vi "Read - Asynchronous.vi"(8 "error in":errorcluster, 11 "Serial IO in":refnum<class "Serial IO.lvclass">) -> (0 "error out":errorcluster, 2 "read buffer":string, 3 "Serial IO out":refnum<class "Serial IO.lvclass">)   [LabVIEW 2015, in "Serial IO.lvclass"]
doc: "Read asynchronously from the serial port. Requires no prior write."
uses:
  Serial IO.lvclass
  Serial IO.lvclass/Serial IO.ctl
  <vilib>/Platform/TimedLoop/XDataNode/timing_clust.ctl
  <vilib>/Platform/TimedLoop/XDataNode/nitl_modes.ctl
  <vilib>/Platform/TimedLoop/XDataNode/wakeup.ctl
  <vilib>/Platform/TimedLoop/XDataNode/XDataNode.xnode
  <vilib>/Platform/TimedLoop/XDataNode/XDNodeRunTimeDep.lvlib
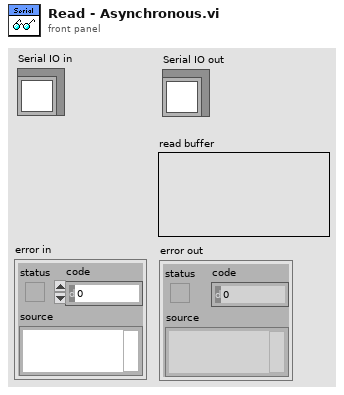
[diagram p1: front panel]
types:
  T1 = typedef "XDNodeRunTimeDep.lvlib/timing_clust.ctl" = cluster{"Expected End [f-1]":u64, "Actual End [f-1]":u64, "Finished Late? [f-1]":bool, "Expected End [i-1]":u64, "Actual End [i-1]":u64, "Finished Late? [i-1]":bool, "Expected Start [i]":u64, "Actual Start [i]":u64, "Expected Start [f]":u64, "Actual Start [f]":u64, "Source Name":string, "Structure Name":string, "Period":i64, "Deadline":i64, "Offset":i64, "Start":i64, "Priority":i32, "Timeout":i32, "Mode":T2, "Wakeup Reason":T3, "Error":errorcluster, "Source Type":string, "Secondary Source Type":string, "Global End Time":u64, "Global Start Time":u64, "Frame Duration":u64, "Iteration Duration":u64, "Assigned CPU":i32, "I/O Scan Engine Mode":u32}
  T2 = typedef "XDNodeRunTimeDep.lvlib/nitl_modes.ctl" = enum32{"No Change", "Process missed periods, maintain original phase", "Discard missed periods, maintain original phase", "Process missed periods, ignore original phase", "Discard missed periods, ignore original phase"}
  T3 = typedef "XDNodeRunTimeDep.lvlib/wakeup.ctl" = enum32{"Normal", "Aborted", "Asynchronous wakeup", "Timing source error", "Timed loop error", "Timeout"}
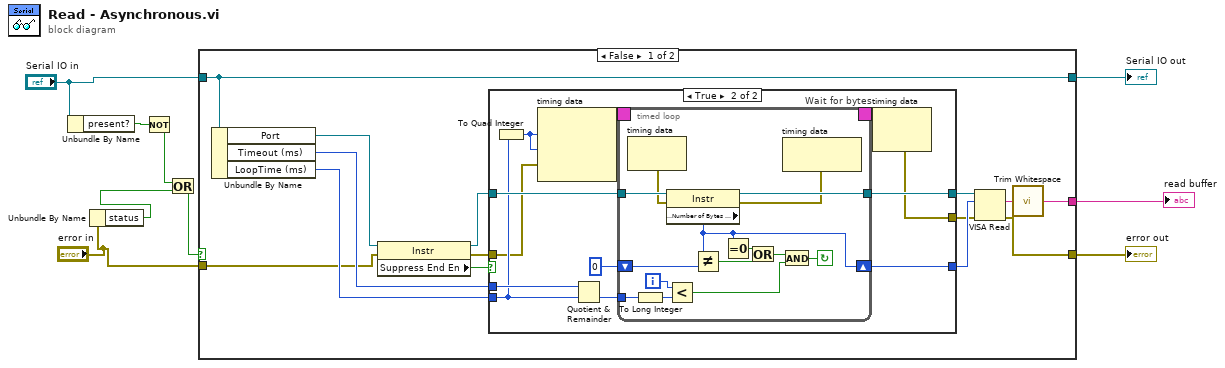
[diagram p0: block diagram]
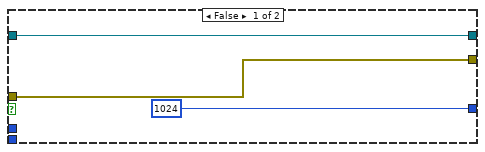
[diagram p2: hidden frame]
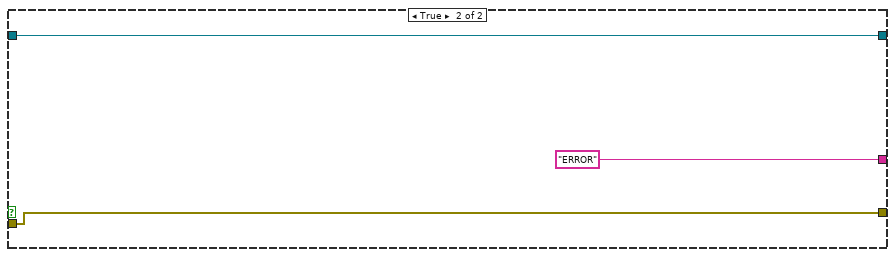
[diagram p3: hidden frame]
diagram:
  n1 = Unbundle By Name("Serial IO in") -> ("present?"=w5:bool)
  n2 = Unbundle By Name("error in") -> ("status"=w3:bool)
  n3 = Not(x=w5) -> (.not. x?=w4:bool)
  n4 = Or(x=w4, y=w3) -> (x .or. y?=w1:bool)
  n5 = case shown="False" w1 {
    tunnel: [w14 w65] -> w9
    tunnel: [w23 w67] -> w8
    tunnel: "Serial IO in" -> [w23 w67]
    tunnel: [w15 "ERROR" ("read buffer")] -> w7
    tunnel: "error in" -> [w10 w65]
    frame False {
      n6 = Unbundle By Name(w23) -> ("Port"=w22:refnum<visa-resource-name>, "Timeout (ms)"=w18:u32, "LoopTime (ms)"=w17:u32)
      n7 = property class="Instr"(reference=w22, error in=w10) -> (reference out=w19:refnum<visa-resource-name>, error out=w20:errorcluster, "Suppress End En"=w21:bool)
      n8 = case shown="True" w21 {
        tunnel: w19 -> [w25 w36]
        tunnel: [w25 w35] -> w13
        tunnel: [u32 1024 w34] -> w12
        tunnel: w18 -> [_ w33]
        tunnel: w17 -> [_ w32]
        tunnel: w20 -> [w26 w31]
        tunnel: [w26 w30] -> w11
        frame False {
        }
        frame True {
          n9 = To Quad Integer(1:w32) -> (0:w27:i64)
          n10 = node-c288(w27, w27, w31) -> (w38:T1)
          n11 = Quotient & Remainder(x=w33, y=w32) -> (floor(x/y)=w29:u32)  [unwired: 1 out]
          n12 = timed-loop "Wait for bytes" {
            tunnel: w36 -> [w52]
            tunnel: [w51] -> w35
            tunnel: w29 -> [w40]
            shift-right: [w43] -> w34
            shift-left: u32 0 -> [w44]
            timing: w38 -> [_]
            timing-out: [_] -> w37
            i -> [w50]
            stop <- w49 continue-if-true
            n13 = node-c288() -> (w42:errorcluster)  [unwired: 1 in]
            n14 = To Long Integer(number=w40) -> (32bit integer=w39:i32)
            n15 = property class="Instr"(reference=w52, error in=w42) -> (reference out=w51:refnum<visa-resource-name>, error out=w41:errorcluster, "Serial Settings:Number of Bytes at Serial Port"=w43:u32)
            n16 = Less?(x=w50, y=w39) -> (x < y?=w48:bool)
            n17 = Not Equal?(x=w43, y=w44) -> (x != y?=w47:bool)
            n18 = Equal To 0?(x=w43) -> (x = 0?=w46:bool)
            n19 = Or(x=w46, y=w47) -> (x .or. y?=w45:bool)
            n20 = And(x=w45, y=w48) -> (x .and. y?=w49:bool)
            n21 = node-c288(w41) -> ()  [unwired: 1 out]
          }
          n22 = node-c288(w37) -> (w30:errorcluster)
        }
      }
      n23 = VISA Read(VISA resource name=w13, byte count=w12, error in (no error)=w11) -> (read buffer=w16:string, error out=w14:errorcluster)  [unwired: 2 out]
      n24 = call <vilib>:"Trim Whitespace.vi"("string"=w16) -> ("trimmed string"=w15:string)  [unwired: 1 in]
    }
    frame True {
    }
  }
  "error out" <- w9
  "Serial IO out" <- w8
  "read buffer" <- w7
